vi "BMU诊断标定.vi"(5 "timeout":u32, 6 "Socket":dbl, 7 "通用配置?":bool, 8 "CAN端口":u16(ring), 9 "设备索引号":u16(ring), 10 "CAN卡类型":u32(ring)=21, 11 "从板号":u8=1) -> (3 "成功?":bool)   [LabVIEW 2013] (continued)
            tunnel: [w559 _ _] -> w557
            frame #0 {
              n484 = global read "功能码全局.vi" "15"() -> (w584:bool[])
              n485 = global read "功能码全局.vi" "16"() -> (w575:bool[])
              n486 = Index Array(array=w584) -> (element #1=w583:bool, element #2=w581:bool, element #3=w579:bool, element #4=w577:bool, element #5=w582:bool, element #6=w580:bool, element #7=w578:bool, element #8=w576:bool)  [unwired: 8 in]
              n487 = Index Array(array=w575) -> (element #5=w566:bool, element #6=w574:bool, element #7=w565:bool, element #8=w573:bool)  [unwired: 8 in, 4 out]
              n488 = Not Or(1:w573, 2:w574) -> (0:w563:bool)
              n489 = Not Or(1:w565, 2:w566) -> (0:w564:bool)
              n490 = Not Or(1:w582, 2:w583) -> (0:w569:bool)
              n491 = Not Or(1:w580, 2:w581) -> (0:w570:bool)
              n492 = Not Or(1:w578, 2:w579) -> (0:w571:bool)
              n493 = Not Or(1:w576, 2:w577) -> (0:w572:bool)
              n494 = Compound Arithmetic op=OR(w569, w570, w571, w572, w563) -> (w568:bool)
              "从板项目信息" <- w568
              n495 = property class="Tree (严格)"(reference=w561, "Active Item Row Number"=1 ("活动项:行数"), "Disabled?"=w568, "Active Item Row Number"=2 ("活动项:行数"), "Disabled?"=w569, "Active Item Row Number"=3 ("活动项:行数"), "Disabled?"=w570, "Active Item Row Number"=4 ("活动项:行数"), "Disabled?"=w571, "Active Item Row Number"=5 ("活动项:行数"), "Disabled?"=w572, "Active Item Row Number"=0 ("活动项:行数"), "Disabled?"=w564) -> (error out=w560:errorcluster)  [unwired: 1 in, 1 out]
              n496 = for {
                N: 8 -> [_]
                tunnel: w561 -> [w596]
                tunnel: w563 -> [w592]
                tunnel: w560 -> [w591]
                tunnel: [w590] -> w559
                i -> [w594]
                n497 = Add(x=w594, y=6) -> (x+y=w595:i32)
                n498 = property class="Tree (严格)"(reference=w596, error in=w591, "Active Item Row Number"=w595, "Disabled?"=w592) -> (error out=w590:errorcluster)  [unwired: 1 out]
              }
              n499 = call <vilib>:"Clear Errors.vi"("error in (no error)"=w559) -> ()  [unwired: 6 in, 1 out]
            }
            frame #1 {
              w609 = 8
              n500 = global read "功能码全局.vi" "18"() -> (w618:bool[])
              n501 = Index Array(array=w618) -> (element #1=w601:bool, element #2=w602:bool, element #3=w617:bool, element #4=w612:bool, element #5=w606:bool, element #6=w616:bool, element #7=w611:bool, element #8=w605:bool)  [unwired: 8 in]
              n502 = Not Or(1:w602, 2:w601) -> (0:w597:bool)
              n503 = property class="Tree (严格)"(reference=w598, "Active Item Row Number"=46 ("活动项:行数"), "Disabled?"=w597, "Active Item Row Number"=47 ("活动项:行数"), "Disabled?"=w597, "Active Item Row Number"=48 ("活动项:行数"), "Disabled?"=w597) -> ()  [unwired: 1 in, 2 out]
              n504 = Not Or(1:w605, 2:w606) -> (0:w604:bool)
              n505 = Not Or(1:w616, 2:w617) -> (0:w615:bool)
              n506 = Not Or(1:w611, 2:w612) -> (0:w610:bool)
              n507 = for {
                N: w609 -> [_]
                tunnel: w598 -> [w639]
                tunnel: w615 -> [w635]
                tunnel: "error out" -> [w634]
                tunnel: [w633] -> w613
                i -> [w637]
                n508 = Add(x=w637, y=14) -> (x+y=w638:i32)
                n509 = property class="Tree (严格)"(reference=w639, error in=w634, "Active Item Row Number"=w638, "Disabled?"=w635) -> (error out=w633:errorcluster)  [unwired: 1 out]
              }
              n510 = for {
                N: w609 -> [_]
                tunnel: w598 -> [w632]
                tunnel: w610 -> [w628]
                tunnel: w613 -> [w627]
                tunnel: [w626] -> w608
                i -> [w630]
                n511 = Add(x=w630, y=22) -> (x+y=w631:i32)
                n512 = property class="Tree (严格)"(reference=w632, error in=w627, "Active Item Row Number"=w631, "Disabled?"=w628) -> (error out=w626:errorcluster)  [unwired: 1 out]
              }
              n513 = for {
                N: w609 -> [_]
                tunnel: w598 -> [w625]
                tunnel: w604 -> [w621]
                tunnel: w608 -> [w620]
                tunnel: [w619] -> w607
                i -> [w623]
                n514 = Add(x=w623, y=30) -> (x+y=w624:i32)
                n515 = property class="Tree (严格)"(reference=w625, error in=w620, "Active Item Row Number"=w624, "Disabled?"=w621) -> (error out=w619:errorcluster)  [unwired: 1 out]
              }
              n516 = call <vilib>:"Clear Errors.vi"("error in (no error)"=w607) -> ()  [unwired: 6 in, 1 out]
            }
            frame #2 {
              n517 = global read "功能码全局.vi" "23"() -> (w664:bool[])
              n518 = global read "功能码全局.vi" "24"() -> (w662:bool[])
              n519 = Index Array(array=w664) -> (element #3=w663:bool, element #4=w660:bool, element #5=w658:bool, element #6=w656:bool, element #7=w654:bool, element #8=w652:bool)  [unwired: 8 in, 2 out]
              n520 = Index Array(array=w662) -> (element #3=w661:bool, element #4=w659:bool, element #5=w657:bool, element #6=w655:bool, element #7=w653:bool, element #8=w651:bool)  [unwired: 8 in, 2 out]
              n521 = Not Or(1:w661, 2:w663) -> (0:w650:bool)
              n522 = Not Or(1:w659, 2:w660) -> (0:w645:bool)
              n523 = Not Or(1:w657, 2:w658) -> (0:w646:bool)
              n524 = Not Or(1:w655, 2:w656) -> (0:w647:bool)
              n525 = Not Or(1:w653, 2:w654) -> (0:w649:bool)
              n526 = Not Or(1:w651, 2:w652) -> (0:w648:bool)
              n527 = Build Array(w650, w650, w649, w648, w647, w646, w645) -> (w643:bool[])
              n528 = And Array Elements(Boolean array=w643) -> (logical AND=w644:bool)
              n529 = Insert Into Array(array=w643, index=0 ("索引"), new element=w644) -> (w641:bool[])
              n530 = for {
                N: 8 -> [_]
                tunnel: w640 -> [w674]
                tunnel: w641 -> [w670] mode=indexing
                tunnel: errorcluster {"status"=FALSE, "code"=0, "source"=""} ("error out 2") -> [w669]
                tunnel: [w668] -> w666
                i -> [w672]
                n531 = Add(x=w672, y=38) -> (x+y=w673:i32)
                n532 = property class="Tree (严格)"(reference=w674, error in=w669, "Active Item Row Number"=w673, "Disabled?"=w670) -> (error out=w668:errorcluster)  [unwired: 1 out]
              }
              n533 = call <vilib>:"Clear Errors.vi"("error in (no error)"=w666) -> ()  [unwired: 6 in, 1 out]
            }
          }
        }
        frame Enabled {
        }
      }
    }
  }
  n534 = disable-structure shown="禁用" {
    disable-tunnel: w43 -> [w907 _]
    disable-tunnel: w42 -> [w906 w927]
    disable-tunnel: [w905 w927] -> w41
    frame Disabled {
      n535 = stacked-sequence {
        tunnel: [_ _ w915] -> w905
        tunnel: w907 -> [_ _ _]
        tunnel: w906 -> [_ _ w913]
        frame #0 {
          w908 = u32 4 items=["PCI5121"=1, "PCI9810"=2, "USBCAN1"=3, "USBCAN2"=4, "PCI9820"=5, "PCI5110"=7, "CANLite(mini)"=8, "ISA9620"=9, "ISA5420"=10, "PC104CAN"=11, "DNP9810"=13, "PCI9840B"=14, "PC104C2"=15, "PCI9820I"=16, "pec9920"=18, "USBCAN_E_U"=20, "USBCAN_2E_U"=21] ("CAN卡类型")
          n536 = local write "CAN卡类型"(w908) -> ()
        }
        frame #1 {
          n537 = disable-structure shown="禁用" {
            frame Disabled {
              n538 = local read "设备索引号"() -> (w910:u16)
              n539 = local read "CAN卡类型"() -> (w909:u32)
              n540 = local read "CAN端口"() -> (w911:u16)
              n541 = dll-call lib="PTH1abs FBluewave New EnergySVN_WorkAutoTest_TestStandtrunkAutoTest_TestStandDriverZlgCanBHN01è¯»ååæ°data\nkerneldlls\nusbcan.dll" fn="VCI_ClearBuffer"("DeviceType"=w909, "DeviceInd"=w910, "CANInd"=w911) -> (error out=w912:errorcluster)  [unwired: 4 in, 4 out]
              n542 = call <vilib>:"Clear Errors.vi"("error in (no error)"=w912) -> ()  [unwired: 6 in, 1 out]
            }
            frame Enabled {
            }
          }
        }
        frame #2 {
          w922 = u8 0 items=["Normal", "Listen Only"] ("工作方式")
          w921 = u8 1 items=["Dual Filter", "Single Filter"] ("滤波方式")
          n543 = local read "设备索引号"() -> (w917:u16)
          n544 = local read "CAN卡类型"() -> (w916:u32)
          n545 = local read "CAN端口"() -> (w918:u16)
          n546 = call "CAN_Init-8.6.vi"("CAN卡类型"=w916, "设备索引号"=w917, "CAN端口"=w918, "操作类型"=enum16{"初始化CAN", "关闭CAN"}."初始化CAN", "error in (no error)"=w913, "滤波方式"=w921, "Accept Code"=u32 3221225472, "簇"=T23 {"打开CAN"=TRUE, "初始化CAN"=TRUE, "开始CAN"=TRUE, "重启"=FALSE, "关闭CAN"=FALSE}, "Mask Code"=u32 1073741823 ("Accept Code"), "工作方式"=w922, "是否滤波"=TRUE, "滤波选择"=T22 {"fiter_mode"=1, "fiter_endid"=402653184, "fiter_startid"=419430399}) -> ("CAN 操作结果"=→"CAN":bool, "error out"=w915:errorcluster)  [unwired: 2 in, 4 out]
        }
      }
    }
    frame Enabled {
    }
  }
  n547 = call <vilib>:"Open Config Data.vi"("configuration file path"=path "D:/BlueWay/BMU从板号.ini") -> ("refnum"=w45:T19)  [unwired: 8 in, 2 out]
  n548 = call-poly <vilib>:"Read Key.vi"("section"="BMUNO", "key"="BMUNO", "refnum"=w45) -> ("error out"=w34:errorcluster, "value"=w44:string, "refnum out"=w35:T19)  [unwired: 5 in, 1 out]
  n549 = local read "从板号"() -> (w14:u8)
  n550 = Decimal String To Number(string=w44) -> ()  [unwired: 2 in, 2 out]
  n551 = Number To Decimal String(number="Socket") -> (decimal integer string=w10:string)  [unwired: 1 in]
  n552 = Concatenate Strings("CMD" ("名称（未命名）"), w10) -> (w2:string)
  n553 = local write "从板号"(w14) -> ()
  n554 = local read "Socket"() -> (w9:dbl)
  n555 = Number To Decimal String(number=w9) -> (decimal integer string=w6:string)  [unwired: 1 in]
  n556 = Obtain Queue(name (unnamed)=w2, element data type=w2, error in (no error)=w41) -> (queue out=w79:refnum<queue>, error out=w50:errorcluster)  [unwired: 2 in, 1 out]
  n557 = Concatenate Strings("read" ("名称（未命名）"), w6) -> (w7:string)
  "连接的字符串" <- w7
  n558 = Obtain Queue(name (unnamed)=w7, element data type="读参数") -> (queue out=w73:refnum<queue>, error out=w72:errorcluster)  [unwired: 3 in, 1 out]
  n559 = call-poly <vilib>:"Read Key.vi"("section"="CURRBMUNO", "error in (no error)"=w34, "key"="CURRBMUNO", "refnum"=w35) -> ("error out"=w30:errorcluster, "value"=w40:string, "refnum out"=w31:T19)  [unwired: 4 in, 1 out]
  n560 = call-poly <vilib>:"Read Key.vi"("section"="CONFIGTYPE", "error in (no error)"=w30, "key"="CONFIGTYPE", "refnum"=w31) -> ("error out"=w26:errorcluster, "value"=w29:string, "refnum out"=w25:T19)  [unwired: 4 in, 1 out]
  n561 = call-poly <vilib>:"Read Key.vi"("section"="BMUSERIAL", "error in (no error)"=w26, "default value"="60", "key"="BMUSERIAL", "refnum"=w25) -> ("error out"=w20:errorcluster, "value"=w23:string, "refnum out"=w22:T19)  [unwired: 3 in, 1 out]
  n562 = call-poly <vilib>:"Read Key.vi"("section"=w18, "error in (no error)"=w20, "default value"="BNET0001", "key"=w18, "refnum"=w22) -> ("error out"=w19:errorcluster, "value"=w16:string, "refnum out"=w21:T19)  [unwired: 3 in, 1 out]
  n563 = Decimal String To Number(string=w40) -> ()  [unwired: 2 in, 2 out]
  n564 = call <vilib>:"Obtain Semaphore Reference.vi"("name (unnamed)"=w2) -> ("semaphore"=w1:T24)  [unwired: 4 in, 2 out]
  n565 = local write "二维码"(w16) -> ()
  n566 = call <vilib>:"Close Config Data.vi"("error in (no error)"=w19, "refnum"=w21) -> ()  [unwired: 8 in, 2 out]
  n567 = local write "失败？"(TRUE ("失败")) -> ()
  n568 = local write "timeout"(FALSE ("timeout")) -> ()
  n569 = local write "成功?"(FALSE ("成功?")) -> ()
  n570 = local read "从板号"() -> (w13:u8)
  n571 = local write "停止"(FALSE ("停止")) -> ()
  n572 = Tick Count (ms)() -> (millisecond timer value=w4:u32)
  n573 = while {
    tunnel: w73 -> [w940]
    tunnel: w72 -> [w939]
    tunnel: w13 -> [w934]
    tunnel: w1 -> [w929]
    stop <- w930 stop-if-true
    n574 = local read "停止"() -> (w931:bool)
    n575 = global read "全局 1.vi" "名称"() -> (w933:string)
    n576 = local read "控制1"() -> (w936:bool)
    n577 = local read "timeout"() -> (w932:bool)
    n578 = Dequeue Element(queue=w940, timeout in ms (-1)=50 ("超时毫秒(-1)"), error in (no error)=w939) -> (element=w938:T3, error out=w928:errorcluster)  [unwired: 2 out]
    n579 = Or(x=w932, y=w931) -> (x .or. y?=w930:bool)
    n580 = case shown="无错误" w928 {
      tunnel: w938 -> [w948 _]
      tunnel: "写?" -> [w945 _]
      tunnel: w936 -> [w944 _]
      tunnel: w934 -> [w943 _]
      tunnel: w933 -> [w942 _]
      tunnel: w929 -> [w941 _]
      frame No Error {
        n581 = Unbundle(w948) -> ("return type"=w947:u32, "pReceive"=w946:T25)
        n582 = for {
          N: w947 -> [_]
          tunnel: w946 -> [w955] mode=indexing
          tunnel: w945 -> [w953]
          tunnel: w944 -> [w952]
          tunnel: w943 -> [w951]
          tunnel: w942 -> [w950]
          tunnel: w941 -> [w949]
          n583 = Unbundle By Name(w955) -> ("ID"=w956:u32)
          n584 = call "ID解析.vi"("ID"=w956) -> ("PDU(1)"=w954:i32)  [unwired: 10 out]
          n585 = case shown="18" w954 {
            tunnel: w955 -> [_ w969]
            tunnel: w953 -> [_ w961]
            tunnel: w952 -> [_ w960]
            tunnel: w951 -> [_ w959]
            tunnel: w950 -> [_ w958]
            tunnel: w949 -> [_ w957]
            frame 0, Default {
            }
            frame 24 {
              n586 = local read "主从选择"() -> (w962:enum32{"主板", "从板"})
              n587 = local read "设备索引号"() -> (w965:u16)
              n588 = local read "CAN卡类型"() -> (w964:u32)
              n589 = local read "CAN端口"() -> (w966:u16)
              n590 = case shown="\"从板\"" w962 {
                tunnel: [0 ("FUNC") w972] -> w963
                tunnel: w959 -> [_ w973]
                tunnel: w958 -> [_ w971]
                frame "主板", Default {
                }
                frame "从板" {
                  n591 = local read "从板号"() -> (w974:u8)
                  n592 = Equal?(x=w971, y="从板号") -> (x = y?=w975:bool)
                  n593 = Select(t=w973, s=w975, f=w974) -> (s? t:f=w972:u8)
                }
              }
              n594 = disable-structure shown="禁用" {
                disable-tunnel: w969 -> [w977 _]
                frame Disabled {
                  n595 = call "标定授权读取.vi"("VCI_Receive"=w977) -> ()  [unwired: 1 out]
                }
                frame Enabled {
                }
              }
              n596 = local read "面板选择"() -> (w968:T7)
              n597 = case shown="\"读写参数\", 默认" w968 {
                tunnel: w961 -> [w985 _ _ _]
                tunnel: "命令" -> [w986 w1090 w1345 w1485]
                tunnel: w962 -> [w995 _ w1353 w1493]
                tunnel: w969 -> [_ _ _ _]
                tunnel: w969 -> [w991 w1091 w1347 w1487]
                tunnel: w966 -> [w990 w1092 w1348 w1488]
                tunnel: w965 -> [w989 w1093 w1349 w1489]
                tunnel: w964 -> [w988 w1094 w1350 w1490]
                tunnel: w963 -> [w987 _ w1346 w1486]
                tunnel: w960 -> [w981 _ _ _]
                tunnel: w957 -> [w980 _ _ _]
                frame "读写参数", Default {
                  n598 = control-ref of="流控帧 2"() -> (w978:refnum<vi>)
                  n599 = control-ref of="流控帧"() -> (w979:refnum<vi>)
                  n600 = local read "命令序号"() -> (w984:u8)
                  n601 = call "多帧接收机制(EV05).vi"("can卡类型"=w988, "设备索引号"=w989, "CAN端口"=w990, "VCI_Receive"=w991, "命令"=w986, "板号"=w987, "流控帧"=w979, "写?"=w985, "流控帧2"=w978, "命令序号"=w984) -> ("错误信号"=w982:bool, "错误代码"=w994:i32, "输出数组"=w993:u8[], "读错误代码"=w983:u8[], "结束信号"=w992:bool)  [unwired: 5 out]
                  n602 = case shown="真" w985 {
                    tunnel: w992 -> [w1005 w1070]
                    tunnel: w994 -> [w1004 w1069]
                    tunnel: w984 -> [w1003 _]
                    tunnel: w993 -> [w1002 _]
                    tunnel: w986 -> [w1001 _]
                    tunnel: w995 -> [w999 w1068]
                    tunnel: w983 -> [w998 _]
                    tunnel: w982 -> [w997 _]
                    tunnel: w981 -> [w996 _]
                    tunnel: w980 -> [_ w1064]
                    frame False {
                      # "读参数"
                      n603 = And(x=w996, y=w1005) -> (x .and. y?=w1000:bool)
                      n604 = case shown="真" w1000 {
                        tunnel: w1004 -> [_ w1016]
                        tunnel: w1003 -> [_ w1015]
                        tunnel: w1002 -> [_ w1014]
                        tunnel: w1001 -> [_ w1013]
                        tunnel: w999 -> [_ w1009]
                        tunnel: w998 -> [_ w1007]
                        tunnel: w997 -> [_ w1008]
                        frame False {
                        }
                        frame True {
                          n605 = case shown="假" w1008 {
                            tunnel: w1016 -> [w1026 _]
                            tunnel: w1015 -> [w1025 _]
                            tunnel: w1014 -> [w1024 _]
                            tunnel: w1013 -> [w1022 _]
                            tunnel: w1009 -> [w1018 _]
                            tunnel: w1007 -> [_ w1052]
                            frame False {
                              n606 = case shown="\"从板\"" w1018 {
                                tunnel: [w1027 _] -> w1021
                                tunnel: [_ w1040] -> w1020
                                frame "主板", Default {
                                n607 = stacked-sequence {
                                tunnel: [_ w1039] -> w1027
                                frame #0 {
                                n608 = control-ref of="一级故障"() -> (w1033:refnum<vi>)
                                n609 = control-ref of="一级故障 2"() -> (w1035:refnum<vi>)
                                n610 = control-ref of="一级故障 3"() -> (w1036:refnum<vi>)
                                n611 = control-ref of="加热控制参数"() -> (w1037:refnum<vi>)
                                n612 = control-ref of="充电控制参数"() -> (w1038:refnum<vi>)
                                n613 = control-ref of="电池信息"() -> (w1031:refnum<vi>)
                                n614 = control-ref of="项目信息"() -> (w1034:refnum<vi>)
                                n615 = control-ref of="项目信息2"() -> (w1032:refnum<vi>)
                                n616 = control-ref of="高压参数"() -> (w1030:refnum<vi>)
                                n617 = local read "主板数据"() -> (w1029:T4)
                                n618 = Bundle(cluster=w1029, "项目信息"=w1034, "一级故障 4"=w1032, "一级故障"=w1033, "一级故障 2"=w1035, "一级故障 3"=w1036, "加热控制参数"=w1037, "充电控制参数"=w1038, "高压参数"=w1030, "电池信息"=w1031) -> (w1028:T4)
                                n619 = local write "主板数据"(w1028) -> ()
                                }
                                frame #1 {
                                n620 = control-ref of="主板数据"() -> (w1039:refnum<vi>)
                                }
                                }
                                }
                                frame "从板" {
                                n621 = stacked-sequence {
                                tunnel: [_ w1051] -> w1040
                                frame #0 {
                                n622 = control-ref of="从板号"() -> (w1045:refnum<vi>)
                                n623 = control-ref of="项目信息 2"() -> (w1046:refnum<vi>)
                                n624 = control-ref of="电池组信息"() -> (w1044:refnum<vi>)
                                n625 = control-ref of="加热控制参数"() -> (w1047:refnum<vi>)
                                n626 = control-ref of="一级故障(从板)"() -> (w1048:refnum<vi>)
                                n627 = control-ref of="二级故障(从板)"() -> (w1049:refnum<vi>)
                                n628 = control-ref of="三级故障(从板)"() -> (w1050:refnum<vi>)
                                n629 = control-ref of="均衡参数"() -> (w1043:refnum<vi>)
                                n630 = local read "从板信息"() -> (w1042:T2)
                                n631 = Bundle(cluster=w1042, "从板号"=w1045, "项目信息 2"=w1046, "加热控制参数"=w1047, "一级故障(从板)"=w1048, "二级故障(从板)"=w1049, "三级故障(从板)"=w1050, "电池组信息(从板)"=w1044, "均衡参数"=w1043) -> (w1041:T2)
                                n632 = local write "从板信息"(w1041) -> ()
                                }
                                frame #1 {
                                n633 = control-ref of="从板信息"() -> (w1051:refnum<vi>)
                                }
                                }
                                }
                              }
                              n634 = control-ref of="结果"() -> (w1023:refnum<vi>)
                              n635 = control-ref of="从板个数"() -> (w1019:refnum<vi>)
                              n636 = control-ref of="二维码"() -> (w1017:refnum<vi>)
                              n637 = call "输出数据解析.vi"("主板引用"=w1021, "错误代码"=w1026, "命令序号"=w1025, "输入数组"=w1024, "命令"=w1022, "从板引用"=w1020, "进度引用"=w1023, "板选择"=w1018, "从板个数"=w1019, "从板二维码信息"=w1017) -> ()  [unwired: 6 in, 4 out]
                            }
                            frame True {
                              n638 = Index Array(array=w1052, index #1=0 ("索引"), index #2=1 ("索引")) -> (element #1=w1055:u8, element #2=w1056:u8)
                              n639 = Join Numbers(hi=w1055, lo=w1056) -> ((hi.lo)=w1054:u16)
                              n640 = Number To Hexadecimal String(2:w1054) -> (0:w1053:string)  [unwired: 1 out]
                              n641 = control-ref of="结果"() -> (w1061:refnum<vi>)
                              n642 = Concatenate Strings("0x" ("字符串"), w1053) -> (w1062:string)
                              n643 = Build Array(w1062) -> (w1063:string[])
                              n644 = call "表格编辑.vi"("新元素/子数组"=w1063, "活动单元格:单元格背景色"=u32 16740749, "MCListbox引用句柄"=w1061) -> ()  [unwired: 9 out]
                            }
                          }
                          n645 = global write "EV05全局变量1.vi" "流控帧 2"(FALSE ("流控帧 2")) -> ()
                          n646 = global write "EV05全局变量1.vi" "输出数组"(i32[] []) -> ()
                          n647 = local write "控制1"(FALSE ("控制1")) -> ()
                          n648 = local write "消除"(FALSE ("消除")) -> ()
                        }
                      }
                    }
                    frame True {
                      # "写参数判定"
                      n649 = And(x="控制1", y=w1070) -> (x .and. y?=w1067:bool)
                      n650 = case shown="真" w1067 {
                        tunnel: w1069 -> [_ w1080]
                        tunnel: w1068 -> [_ w1077]
                        tunnel: w1064 -> [_ w1072]
                        frame False {
                        }
                        frame True {
                          n651 = call <vilib>:"Unset Busy.vi"() -> ()  [unwired: 2 in, 10 out]
                          n652 = case shown="\"从板\"" w1077 {
                            tunnel: [w1081 w1082] -> w1079
                            frame "主板", Default {
                              n653 = local read "主板选项"() -> (w1081:string)
                            }
                            frame "从板" {
                              n654 = local read "从板选项"() -> (w1082:string)
                            }
                          }
                          n655 = control-ref of="结果"() -> (w1078:refnum<vi>)
                          n656 = local read "Socket"() -> (w1073:dbl)
                          n657 = call "输入数据判定.vi"("semaphore"=w1072, "Socket"=w1073, "主从选择"=w1077, "主板选项"=w1079, "进度引用"=w1078, "错误代码"=w1080) -> ("读取超时"=→"读取超时":bool)  [unwired: 1 in, 4 out]
                          n658 = global write "EV05全局变量1.vi" "流控帧 2"(FALSE ("流控帧 2")) -> ()
                          n659 = local write "控制1"(FALSE ("控制1")) -> ()
                          n660 = local write "消除"(FALSE ("消除")) -> ()
                        }
                      }
                      n661 = global write "EV05全局变量1.vi" "输出数组"(i32[] []) -> ()
                    }
                  }
                }
                frame "版本读取" {
                  n662 = local read "命令序号"() -> (w1083:u8)
                  n663 = local read "从板板号"() -> (w1086:u8)
                  n664 = local read "控制1"() -> (w1087:bool)
                  n665 = call "多帧接收机制(EV05).vi"("can卡类型"=w1094, "设备索引号"=w1093, "CAN端口"=w1092, "VCI_Receive"=w1091, "命令"=w1090, "板号"=w1086, "命令序号"=w1083) -> ("错误信号"=w1084:bool, "输出数组"=w1095:u8[], "读错误代码"=w1085:u8[], "结束信号"=w1089:bool)  [unwired: 3 in, 6 out]
                  n666 = And(x=w1087, y=w1089) -> (x .and. y?=w1088:bool)
                  n667 = case shown="真" w1088 {
                    tunnel: w1095 -> [_ w1103]
                    tunnel: w1083 -> [_ w1102]
                    tunnel: w1090 -> [_ w1101]
                    tunnel: w1085 -> [_ w1097]
                    tunnel: w1084 -> [_ w1096]
                    frame False {
                    }
                    frame True {
                      n668 = case shown="假" w1096 {
                        tunnel: w1103 -> [w1107 _]
                        tunnel: w1102 -> [w1106 _]
                        tunnel: w1101 -> [w1105 _]
                        tunnel: w1097 -> [w1104 w1331]
                        frame False {
                          n669 = case shown="89" w1105 {
                            tunnel: w1106 -> [_ w1110]
                            tunnel: w1107 -> [_ w1109]
                            tunnel: w1104 -> [_ _]
                            frame 0, Default {
                            }
                            frame 137 {
                              n670 = case shown="1" w1110 {
                                tunnel: w1109 -> [_ w1138 w1182 w1202 w1329]
                                frame 0, Default {
                                }
                                frame 1 {
                                w1120 = "." ("字符串")
                                n671 = Array Subset(array=w1138, index=0 ("索引"), length=14 ("长度")) -> (w1151:u8[])
                                n672 = Index Array(array=w1138, index=14 ("索引")) -> (element=w1141:u8)
                                n673 = Index Array(array=w1138, index #1=15 ("索引"), index #2=16 ("索引")) -> (element #1=w1147:u8, element #2=w1148:u8)
                                n674 = Index Array(array=w1138, index #1=17 ("索引"), index #2=18 ("索引")) -> (element #1=w1142:u8, element #2=w1143:u8)
                                n675 = call "数组去零.vi"("输入"=w1151) -> ("输出"=w1126:dbl[])
                                n676 = Join Numbers(hi=w1142, lo=w1143) -> ((hi.lo)=w1139:u16)
                                n677 = Join Numbers(hi=w1147, lo=w1148) -> ((hi.lo)=w1140:u16)
                                n678 = Number To Decimal String(number=w1141) -> (decimal integer string=w1133:string)  [unwired: 1 out]
                                n679 = Byte Array To String(unsigned byte array=w1126) -> (string=w1125:string)
                                n680 = Number To Decimal String(number=w1139) -> (decimal integer string=w1121:string)  [unwired: 1 out]
                                n681 = Number To Decimal String(number=w1140) -> (decimal integer string=w1132:string)  [unwired: 1 out]
                                n682 = Array Subset(array=w1138, index=21 ("索引"), length=7 ("长度")) -> (w1135:u8[])
                                n683 = Concatenate Strings("V" ("字符串"), w1133, w1120, w1132, w1120, w1121) -> (w1130:string)
                                n684 = call "数组去零.vi"("输入"=w1135) -> ("输出"=w1118:dbl[])
                                n685 = Byte Array To String(unsigned byte array=w1118) -> (string=w1116:string)
                                n686 = call <vilib>:"Space Constant.vi"() -> ("String"=w1117:string)
                                n687 = Equal?(x=w1116, y=w1117) -> (x = y?=w1122:bool)
                                n688 = Concatenate Strings("-" ("字符串"), w1116) -> (w1123:string)
                                n689 = Select(t=w1117, s=w1122, f=w1123) -> (s? t:f=w1119:string)
                                n690 = Concatenate Strings(w1125, "-" ("字符串"), w1130, w1119) -> (w1112:string)
                                n691 = local read "项目软件版本"() -> (w1114:string[])
                                n692 = local read "从板板号"() -> (w1111:u8)
                                n693 = local write "项目软件版本号"(w1112) -> ()
                                n694 = Replace Array Subset(array=w1114, new element=w1112, index=w1111) -> (w1113:string[])
                                n695 = control-ref of="结果"() -> (w1129:refnum<vi>)
                                n696 = local write "项目软件版本"(w1113) -> ()
                                n697 = Build Array("项目软件版本     读取完成" ("读取结果")) -> (w1127:string[])
                                n698 = call "表格编辑(版本读取).vi"("新元素/子数组"=w1127, "活动单元格:单元格背景色"=u32 6618880, "MCListbox引用句柄"=w1129) -> ()  [unwired: 9 out]
                                }
                                frame 2 {
                                w1165 = ""
                                w1162 = "." ("字符串")
                                n699 = Array Subset(array=w1182, index=0 ("索引"), length=14 ("长度")) -> (w1170:u8[])
                                n700 = Index Array(array=w1182, index=14 ("索引")) -> (element=w1185:u8)
                                n701 = Index Array(array=w1182, index #1=15 ("索引"), index #2=16 ("索引")) -> (element #1=w1191:u8, element #2=w1192:u8)
                                n702 = Index Array(array=w1182, index #1=17 ("索引"), index #2=18 ("索引")) -> (element #1=w1186:u8, element #2=w1187:u8)
                                n703 = Join Numbers(hi=w1186, lo=w1187) -> ((hi.lo)=w1183:u16)
                                n704 = Join Numbers(hi=w1191, lo=w1192) -> ((hi.lo)=w1184:u16)
                                n705 = Number To Decimal String(number=w1183) -> (decimal integer string=w1163:string)  [unwired: 1 out]
                                n706 = call "数组去零.vi"("输入"=w1170) -> ("输出"=w1169:dbl[])
                                n707 = Number To Decimal String(number=w1185) -> (decimal integer string=w1177:string)  [unwired: 1 out]
                                n708 = Number To Decimal String(number=w1184) -> (decimal integer string=w1176:string)  [unwired: 1 out]
                                n709 = Array Subset(array=w1182, index=21 ("索引"), length=7 ("长度")) -> (w1179:u8[])
                                n710 = Byte Array To String(unsigned byte array=w1169) -> (string=w1164:string)
                                n711 = call "数组去零.vi"("输入"=w1179) -> ("输出"=w1161:dbl[])
                                n712 = Concatenate Strings("V" ("字符串"), w1177, w1162, w1176, w1162, w1163) -> (w1174:string)
                                n713 = Byte Array To String(unsigned byte array=w1161) -> (string=w1159:string)
                                n714 = Equal?(x=w1165, y=w1159) -> (x = y?=w1166:bool)
                                n715 = Concatenate Strings("-" ("字符串"), w1159) -> (w1167:string)
                                n716 = Select(t=w1165, s=w1166, f=w1167) -> (s? t:f=w1160:string)
                                n717 = Concatenate Strings(w1164, "-" ("字符串"), w1174, w1160) -> (w1155:string)
                                n718 = local read "平台软件版本"() -> (w1157:string[])
                                n719 = local read "从板板号"() -> (w1154:u8)
                                n720 = local write "平台软件版本号"(w1155) -> ()
                                n721 = Replace Array Subset(array=w1157, new element=w1155, index=w1154) -> (w1156:string[])
                                n722 = control-ref of="结果"() -> (w1172:refnum<vi>)
                                n723 = local write "平台软件版本"(w1156) -> ()
                                n724 = Build Array("平台软件版本     读取完成" ("读取结果")) -> (w1171:string[])
                                n725 = call "表格编辑(版本读取).vi"("新元素/子数组"=w1171, "活动单元格:单元格背景色"=u32 6618880, "MCListbox引用句柄"=w1172) -> ()  [unwired: 1 in, 8 out]
                                }
                                frame 3 {
                                n726 = Index Array(array=w1202, index #1=0 ("索引"), index #2=1 ("索引")) -> (element #1=w1198:u8, element #2=w1199:u8)
                                n727 = Join Numbers(hi=w1198, lo=w1199) -> ((hi.lo)=w1197:u16)
                                n728 = case shown="99, 默认" w1197 {
                                tunnel: w1202 -> [w1205 _ w1239]
                                tunnel: w1197 -> [_ _ w1217]
                                frame 0 {
                                n729 = Index Array(array=w1205, index #1=2 ("索引"), index #2=3 ("索引")) -> (element #1=w1209:u8, element #2=w1208:u8)
                                n730 = Join Numbers(hi=w1209, lo=w1208) -> ((hi.lo)=w1204:u16)
                                n731 = for {
                                N: w1204 -> [_]
                                tunnel: w1205 -> [w1214]
                                tunnel: [w1210] -> w1203 mode=indexing
                                i -> [w1213]
                                n732 = Add(x=w1213, y=4) -> (x+y=w1211:i32)
                                n733 = Index Array(array=w1214, index=w1211) -> (element=w1210:u8)
                                }
                                "MODEL号" <- w1203
                                }
                                frame 99, Default {
                                }
                                frame 1..40 {
                                w1222 = ""
                                w1243 = "." ("字符串")
                                n734 = Array Subset(array=w1239, index=2 ("索引"), length=14 ("长度")) -> (w1228:u8[])
                                n735 = Index Array(array=w1239, index=16 ("索引")) -> (element=w1251:u8)
                                n736 = Index Array(array=w1239, index #1=17 ("索引"), index #2=18 ("索引")) -> (element #1=w1257:u8, element #2=w1258:u8)
                                n737 = Index Array(array=w1239, index #1=19 ("索引"), index #2=20 ("索引")) -> (element #1=w1252:u8, element #2=w1253:u8)
                                n738 = Join Numbers(hi=w1252, lo=w1253) -> ((hi.lo)=w1249:u16)
                                n739 = Join Numbers(hi=w1257, lo=w1258) -> ((hi.lo)=w1250:u16)
                                n740 = Number To Decimal String(number=w1217) -> (decimal integer string=w1237:string)  [unwired: 1 out]
                                n741 = Number To Decimal String(number=w1251) -> (decimal integer string=w1245:string)  [unwired: 1 out]
                                n742 = call "数组去零.vi"("输入"=w1228) -> ("输出"=w1227:dbl[])
                                n743 = Number To Decimal String(number=w1250) -> (decimal integer string=w1244:string)  [unwired: 1 out]
                                n744 = Number To Decimal String(number=w1249) -> (decimal integer string=w1242:string)  [unwired: 1 out]
                                n745 = Byte Array To String(unsigned byte array=w1227) -> (string=w1229:string)
                                n746 = Concatenate Strings("第" ("读取结果"), w1237, "模块" ("字符串"), "     读取完成" ("读取结果")) -> (w1230:string)
                                n747 = Concatenate Strings("V" ("字符串"), w1245, w1243, w1244, w1243, w1242) -> (w1240:string)
                                n748 = control-ref of="结果"() -> (w1233:refnum<vi>)
                                n749 = Array Subset(array=w1239, index=23 ("索引"), length=7 ("长度")) -> (w1226:u8[])
                                n750 = call "数组去零.vi"("输入"=w1226) -> ("输出"=w1221:dbl[])
                                n751 = Byte Array To String(unsigned byte array=w1221) -> (string=w1218:string)
                                n752 = Build Array(w1230) -> (w1232:string[])
                                n753 = control-ref of="模块软件版本 2"() -> (w1234:refnum<vi>)
                                n754 = local read "模块软件版本"() -> (w1235:T1)
                                n755 = Equal?(x=w1222, y=w1218) -> (x = y?=w1223:bool)
                                n756 = call "表格编辑(版本读取).vi"("新元素/子数组"=w1232, "活动单元格:单元格背景色"=u32 6618880, "MCListbox引用句柄"=w1233) -> ()  [unwired: 1 in, 8 out]
                                n757 = Concatenate Strings("-" ("字符串"), w1218) -> (w1224:string)
                                n758 = Select(t=w1222, s=w1223, f=w1224) -> (s? t:f=w1220:string)
                                n759 = Concatenate Strings(w1229, "-" ("字符串"), w1240, w1220) -> (w1219:string)
                                n760 = case shown="30" w1217 {
                                tunnel: [_ "VERSIONM" "BCUMCAL" "BMUMCAL" "BMURMCAL" "BCUCMCAL" "BCUDMCAL" "SCH" "BSW" "CDD" "DATALAYER" "DATAANALYSIS" "SOC" "SOH" "SOF" "INTRES" "INTCAN" "CARCAN" "CHGCANL" "THM" "CHGM" "HVM" "LVM" "BALM" "SAFEM" "RUNMODEM" "RELAY" "DO" "GBCHGDET" "SUPPLYPOWGDET" "SUMVDET" "CURDET" "TEMPERDET" "CELLVDET" "ISODET" "AI" "DI" "SYSCONF" "ECUCONF"] -> w1216
                                frame 0, Default {
                                }
                                frame 1 {
                                }
                                frame 2 {
                                }
                                frame 3 {
                                }
                                frame 4 {
                                }
                                frame 5 {
                                }
                                frame 6 {
                                }
                                frame 7 {
                                }
                                frame 8 {
                                }
                                frame 9 {
                                }
                                frame 10 {
                                }
                                frame 11 {
                                }
                                frame 12 {
                                }
                                frame 13 {
                                }
                                frame 14 {
                                }
                                frame 15 {
                                }
                                frame 16 {
                                }
                                frame 17 {
                                }
                                frame 18 {
                                }
                                frame 19 {
                                }
                                frame 20 {
                                }
                                frame 21 {
                                }
                                frame 22 {
                                }
                                frame 23 {
                                }
                                frame 24 {
                                }
                                frame 25 {
                                }
                                frame 26 {
                                }
                                frame 27 {
                                }
                                frame 28 {
                                }
                                frame 29 {
                                }
                                frame 30 {
                                }
                                frame 31 {
                                }
                                frame 32 {
                                }
                                frame 33 {
                                }
                                frame 34 {
                                }
                                frame 35 {
                                }
                                frame 36 {
                                }
                                frame 37 {
                                }
                                frame 38 {
                                }
                                }
                                n761 = case shown="\"全部读取\"" w1235 {
                                tunnel: w1219 -> [w1302 w1310]
                                tunnel: w1217 -> [w1306 w1315]
                                tunnel: w1234 -> [w1308 w1316]
                                tunnel: w1216 -> [w1307 w1314]
                                frame "全部读取" {
                                n762 = Number To Decimal String(number=w1306) -> (decimal integer string=w1305:string)  [unwired: 1 out]
                                n763 = Concatenate Strings(w1305, "-" ("元素"), w1307) -> (w1303:string)
                                n764 = Build Array(w1303, w1302) -> (w1301:string[])
                                n765 = call "表格编辑(模块版本).vi"("新元素/子数组"=w1301, "MCListbox引用句柄"=w1308) -> ()  [unwired: 1 in, 9 out]
                                }
                                frame "BCUMCAL", Default {
                                n766 = Number To Decimal String(number=w1315) -> (decimal integer string=w1313:string)  [unwired: 1 out]
                                n767 = Concatenate Strings(w1313, "-" ("元素"), w1314) -> (w1311:string)
                                n768 = Build Array(w1311, w1310) -> (w1309:string[])
                                n769 = call "表格编辑(模块版本).vi"("新元素/子数组"=w1309, "MCListbox引用句柄"=w1316) -> ()  [unwired: 1 in, 9 out]
                                }
                                }
                                }
                                }
                                }
                                frame 4 {
                                n770 = Array Subset(array=w1329, length=12 ("长度")) -> (w1327:u8[])  [unwired: 1 in]
                                n771 = Byte Array To String(unsigned byte array=w1327) -> (string=w1326:string)
                                n772 = call <vilib>:"Trim Whitespace.vi"("string"=w1326) -> ("trimmed string"=w1318:string)  [unwired: 1 in]
                                n773 = local read "从板板号"() -> (w1317:u8)
                                n774 = local write "硬件版本号"(w1318) -> ()
                                n775 = local read "硬件版本"() -> (w1319:string[])
                                n776 = Replace Array Subset(array=w1319, new element=w1318, index=w1317) -> (w1320:string[])
                                n777 = local write "硬件版本"(w1320) -> ()
                                n778 = global write "EV05全局变量1.vi" "写入超时"(TRUE ("写入超时")) -> ()
                                n779 = control-ref of="结果"() -> (w1324:refnum<vi>)
                                n780 = Build Array("硬件版本     读取完成" ("读取结果")) -> (w1323:string[])
                                n781 = call "表格编辑(版本读取).vi"("新元素/子数组"=w1323, "活动单元格:单元格背景色"=u32 6618880, "MCListbox引用句柄"=w1324) -> ()  [unwired: 9 out]
                                }
                              }
                              n782 = global write "EV05全局变量1.vi" "写入超时"(TRUE ("写入超时")) -> ()
                            }
                          }
                        }
                        frame True {
                          n783 = Index Array(array=w1331, index #1=0 ("索引"), index #2=1 ("索引")) -> (element #1=w1336:u8, element #2=w1337:u8)
                          n784 = Join Numbers(hi=w1336, lo=w1337) -> ((hi.lo)=w1335:u16)
                          n785 = Number To Hexadecimal String(2:w1335) -> (0:w1334:string)  [unwired: 1 out]
                          n786 = control-ref of="结果"() -> (w1333:refnum<vi>)
                          n787 = Concatenate Strings("0x" ("字符串"), w1334) -> (w1341:string)
                          n788 = Build Array(w1341) -> (w1332:string[])
                          n789 = call "表格编辑(版本读取).vi"("新元素/子数组"=w1332, "活动单元格:单元格背景色"=u32 16740749, "MCListbox引用句柄"=w1333) -> ()  [unwired: 9 out]
                        }
                      }
                      n790 = global write "EV05全局变量1.vi" "流控帧 2"(FALSE ("流控帧 2")) -> ()
                      n791 = local write "控制1"(FALSE ("控制1")) -> ()
                      n792 = local write "消除"(FALSE ("消除")) -> ()
                      n793 = call <vilib>:"Unset Busy.vi"() -> ()  [unwired: 2 in, 10 out]
                    }
                  }
                }
                frame "其它诊断" {
                  n794 = local read "命令序号"() -> (w1343:u8)
                  n795 = call "多帧接收机制(EV05).vi"("can卡类型"=w1350, "设备索引号"=w1349, "CAN端口"=w1348, "VCI_Receive"=w1347, "命令"=w1345, "板号"=w1346, "命令序号"=w1343) -> ("错误代码"=w1352:i32, "输出数组"=w1344:u8[], "读错误代码"=w1342:u8[], "结束信号"=w1351:bool)  [unwired: 3 in, 6 out]
                  n796 = case shown="真" w1351 {
                    tunnel: w1353 -> [_ w1354]
                    tunnel: w1352 -> [_ _]
                    tunnel: w1344 -> [_ w1355]
                    tunnel: w1343 -> [_ w1358]
                    tunnel: w1342 -> [_ w1356]
                    frame False {
                    }
                    frame True {
                      n797 = Insert Into Array(array=w1356, new element=w1355) -> (w1357:u8[])  [unwired: 1 in]
                      n798 = case shown="1" w1358 {
                        tunnel: w1357 -> [_ w1367 w1453]
                        tunnel: w1354 -> [_ _ w1448]
                        frame 0, Default {
                        }
                        frame 1 {
                          n799 = Index Array(array=w1367) -> (element #1=w1366:u8, element #2=w1365:u8, element #3=w1364:u8)  [unwired: 3 in]
                          n800 = Join Numbers(hi=w1365, lo=w1364) -> ((hi.lo)=w1363:u16)
                          n801 = case shown="4" w1366 {
                            tunnel: w1367 -> [_ _ _ _ _ _ _ _ _ _]
                            tunnel: w1363 -> [_ w1370 w1378 w1388 w1398 w1408 w1418 w1428 w1438 _]
                            frame 0, Default {
                              n802 = local write "继电器超时处理"(FALSE ("继电器超时处理")) -> ()
                            }
                            frame 1 {
                              n803 = Equal To 0?(x=w1370) -> (x = 0?=w1369:bool)
                              n804 = local write "正级继电器 12"(w1369) -> ()
                              n805 = case shown="假" w1369 {
                                tunnel: w1370 -> [w1373 _]
                                frame False {
                                n806 = local read "正级继电器"() -> (w1375:bool)
                                n807 = Number To Hexadecimal String(2:w1373) -> (0:w1372:string)  [unwired: 1 out]
                                n808 = local write "继电器超时处理"(TRUE ("继电器超时处理")) -> ()
                                n809 = Not(x=w1375) -> (.not. x?=w1374:bool)
                                n810 = Concatenate Strings("继电器操作失败,0x" ("消息"), w1372) -> ()  [unwired: 1 out]
                                n811 = local write "正级继电器"(w1374) -> ()
                                }
                                frame True {
                                (unwired) "继电器操作成功!\n继电器操作成功!\n继电器操作成功!"
                                }
                              }
                            }
                            frame 2 {
                              n812 = Equal To 0?(x=w1378) -> (x = 0?=w1377:bool)
                              n813 = case shown="假" w1377 {
                                tunnel: w1378 -> [w1384 _]
                                tunnel: [w1382 "继电器操作成功!\n继电器操作成功!\n继电器操作成功!"] -> _
                                frame False {
                                n814 = local read "负级继电器"() -> (w1380:bool)
                                n815 = Number To Hexadecimal String(2:w1384) -> (0:w1383:string)  [unwired: 1 out]
                                n816 = local write "继电器超时处理"(TRUE ("继电器超时处理")) -> ()
                                n817 = Not(x=w1380) -> (.not. x?=w1381:bool)
                                n818 = Concatenate Strings("继电器操作失败,0x" ("消息"), w1383) -> (w1382:string)
                                n819 = local write "负级继电器"(w1381) -> ()
                                }
                                frame True {
                                }
                              }
                              n820 = local write "正级继电器 2"(w1377) -> ()
                            }
                            frame 3 {
                              n821 = Equal To 0?(x=w1388) -> (x = 0?=w1387:bool)
                              n822 = case shown="假" w1387 {
                                tunnel: w1388 -> [w1394 _]
                                tunnel: [w1392 "继电器操作成功!\n继电器操作成功!\n继电器操作成功!"] -> _
                                frame False {
                                n823 = local read "预充电继电器"() -> (w1390:bool)
                                n824 = Number To Hexadecimal String(2:w1394) -> (0:w1393:string)  [unwired: 1 out]
                                n825 = local write "继电器超时处理"(TRUE ("继电器超时处理")) -> ()
                                n826 = Not(x=w1390) -> (.not. x?=w1391:bool)
                                n827 = Concatenate Strings("继电器操作失败,0x" ("消息"), w1393) -> (w1392:string)
                                n828 = local write "预充电继电器"(w1391) -> ()
                                }
                                frame True {
                                }
                              }
                              n829 = local write "正级继电器 3"(w1387) -> ()
                            }
                            frame 4 {
                              n830 = Equal To 0?(x=w1398) -> (x = 0?=w1397:bool)
                              n831 = case shown="假" w1397 {
                                tunnel: w1398 -> [w1404 _]
                                tunnel: [w1402 "继电器操作成功!\n继电器操作成功!\n继电器操作成功!"] -> _
                                frame False {
                                n832 = local read "加热继电器"() -> (w1401:bool)
                                n833 = Number To Hexadecimal String(2:w1404) -> (0:w1403:string)  [unwired: 1 out]
                                n834 = local write "继电器超时处理"(TRUE ("继电器超时处理")) -> ()
                                n835 = Not(x=w1401) -> (.not. x?=w1400:bool)
                                n836 = Concatenate Strings("继电器操作失败,0x" ("消息"), w1403) -> (w1402:string)
                                n837 = local write "加热继电器"(w1400) -> ()
                                }
                                frame True {
                                }
                              }
                              n838 = local write "正级继电器 5"(w1397) -> ()
                            }
                            frame 5 {
                              n839 = Equal To 0?(x=w1408) -> (x = 0?=w1407:bool)
                              n840 = case shown="假" w1407 {
                                tunnel: w1408 -> [w1414 _]
                                tunnel: [w1412 "继电器操作成功!\n继电器操作成功!\n继电器操作成功!"] -> _
                                frame False {
                                n841 = local read "充电继电器"() -> (w1410:bool)
                                n842 = Number To Hexadecimal String(2:w1414) -> (0:w1413:string)  [unwired: 1 out]
                                n843 = local write "继电器超时处理"(TRUE ("继电器超时处理")) -> ()
                                n844 = Not(x=w1410) -> (.not. x?=w1411:bool)
                                n845 = Concatenate Strings("继电器操作失败,0x" ("消息"), w1413) -> (w1412:string)
                                n846 = local write "充电继电器"(w1411) -> ()
                                }
                                frame True {
                                }
                              }
                              n847 = local write "正级继电器 4"(w1407) -> ()
                            }
                            frame 6 {
                              n848 = Equal To 0?(x=w1418) -> (x = 0?=w1417:bool)
                              n849 = local write "正级继电器 6"(w1417) -> ()
                              n850 = case shown="假" w1417 {
                                tunnel: w1418 -> [w1424 _]
                                tunnel: [w1422 "继电器操作成功!\n继电器操作成功!\n继电器操作成功!"] -> _
                                frame False {
                                n851 = local read "风机继电器"() -> (w1420:bool)
                                n852 = Number To Hexadecimal String(2:w1424) -> (0:w1423:string)  [unwired: 1 out]
                                n853 = local write "继电器超时处理"(TRUE ("继电器超时处理")) -> ()
                                n854 = Not(x=w1420) -> (.not. x?=w1421:bool)
                                n855 = Concatenate Strings("继电器操作失败,0x" ("消息"), w1423) -> (w1422:string)
                                n856 = local write "风机继电器"(w1421) -> ()
                                }
                                frame True {
                                }
                              }
                            }
                            frame 7 {
                              n857 = Equal To 0?(x=w1428) -> (x = 0?=w1427:bool)
                              n858 = case shown="假" w1427 {
                                tunnel: w1428 -> [w1433 _]
                                tunnel: [w1431 "继电器操作成功!\n继电器操作成功!\n继电器操作成功!"] -> _
                                frame False {
                                n859 = local read "加热继电器(从)"() -> (w1429:bool)
                                n860 = Number To Hexadecimal String(2:w1433) -> (0:w1432:string)  [unwired: 1 out]
                                n861 = Not(x=w1429) -> (.not. x?=w1430:bool)
                                n862 = Concatenate Strings("继电器操作失败,0x" ("消息"), w1432) -> (w1431:string)
                                n863 = local write "加热继电器(从)"(w1430) -> ()
                                }
                                frame True {
                                n864 = local write "继电器超时处理"(TRUE ("继电器超时处理")) -> ()
                                }
                              }
                              n865 = local write "正级继电器 7"(w1427) -> ()
                            }
                            frame 8 {
                              n866 = Equal To 0?(x=w1438) -> (x = 0?=w1437:bool)
                              n867 = case shown="假" w1437 {
                                tunnel: w1438 -> [w1443 _]
                                tunnel: [w1441 "继电器操作成功!\n继电器操作成功!\n继电器操作成功!"] -> _
                                frame False {
                                n868 = local read "风机继电器(从)"() -> (w1439:bool)
                                n869 = Number To Hexadecimal String(2:w1443) -> (0:w1442:string)  [unwired: 1 out]
                                n870 = Not(x=w1439) -> (.not. x?=w1440:bool)
                                n871 = Concatenate Strings("继电器操作失败,0x" ("消息"), w1442) -> (w1441:string)
                                n872 = local write "风机继电器(从)"(w1440) -> ()
                                }
                                frame True {
                                n873 = local write "继电器超时处理"(TRUE ("继电器超时处理")) -> ()
                                }
                              }
